vi "Test App Broadcast Nested Process Messages.vi"(8 "error in (no error)":errorcluster, 11 "Application Test In":refnum<class "Application Dev Test.lvclass">) -> (0 "error out":errorcluster, 3 "Application Test Out":refnum<class "Application Dev Test.lvclass">)   [LabVIEW 2020, in "Application Dev Test.lvclass"]
uses:
  Application Dev Test.lvclass
  C:/Program Files (x86)/National Instruments/LabVIEW 2020/vi.lib/Astemes/LUnit/Test Case.lvclass
  source/Framework Test Suite/Mock Process/Mock Process.lvclass
  C:/Git/astemes-triarc-framework/source/Framework/Process/Process.lvclass
  source/Framework/Application/Application.lvclass
  source/Framework/Process/Process.lvclass/Process.ctl
  source/Framework/Application/Application.lvclass/Application.ctl
  <vilib>/Astemes/LUnit/Test Case.lvclass/Test Case.ctl
  c27f4279-7cb7-4f54-8dc5-63ff7bac36e5.vi
  76411ce1-69dc-435f-b6fb-e9cd8e6b3fac.vi
  source/Framework/Application/Private/Add Process to Map.vi
  source/Framework/Application/Private/Throw Error If Process Already in App.vi
  source/Framework/Process/Protected/Messaging/Send Message.vi
  source/Framework/Process/Public/Lifecycle/Get Lifecycle State.vi
  source/Framework/Process/Protected/SubVIs/Set Context.vi
  source/Framework/Process/Private/SubVIs/Wait for finish.vi
  source/Framework/Process/Private/SubVIs/Set Lifecycle State.vi
  source/Framework/Broadcast Event Helpers/Execution timer.vi
  <vilib>/Astemes/LUnit/Palette/Pass.vi
  <vilib>/Astemes/LUnit/Palette/Fail.vi
  <vilib>/Astemes/LUnit/Compare Variants.vi
  <vilib>/Astemes/LUnit/Describe Comparison.vi
  <vilib>/Astemes/LUnit/Set Assertion Type.vi
  source/Framework/Application/Public/Get Process.vi
  source/Framework/Process/Private/SubVIs/Handle Debug Data.vi
  <vilib>/Utility/error.llb/Clear Errors.vi
  source/Framework/Process/Public/Lifecycle/Leave Process Loop.vi
  <vilib>/Astemes/LUnit/Add test result.vi
  <vilib>/Astemes/LUnit/Variant to string.vi
  source/Framework/Application/Private/Retrieve Process from App.vi
  source/Framework/Application/Private/Parse Process Name.vi
  source/Framework/Application/Private/Get Process from Map.vi
  source/Framework/Logging/Log Debug.vi
  <vilib>/AdvancedString/1D String Array to Delimited String.vi
  <vilib>/Utility/High Resolution Relative Seconds.vi
  <vilib>/Astemes/LUnit/LUnit Record Assertion Result.vi
  source/Framework/Process/Protected/Messaging/Request Message.vi
  <vilib>/AdvancedString/Delimited String to 1D String Array.vi
  <vilib>/Astemes/LUnit/LUnit Aggregate Assertion Results.vi
  source/Framework/Process/Private/SubVIs/Enqueue Request Message.vi
  <vilib>/Astemes/LUnit/Method Result/LUnit Merge Status.vi
  <vilib>/Astemes/LUnit/LUnit Concatenate result strings.vi
  <vilib>/Utility/error.llb/Error Cluster From Error Code.vi
  source/Framework/Process/Public/Read Name.vi
  source/Framework/Process/Private/SubVIs/Wait for Response Message.vi
  source/Framework/Application/Protected/Get Broadcast Events Recursively.vi
  source/Framework/Broadcast Event Helpers/Dequeue Broadcast Message.vi
  <vilib>/Utility/Data Type/Get Type Information.vi
  <vilib>/Utility/LVClass/Get LV Class Name.vi
  source/Framework/Process/Process.lvclass
  Application Dev Test.lvclass/Application Dev Test.ctl
  C:/Git/astemes-triarc-framework/source/Framework/Base/Base.lvclass
  C:/Git/astemes-triarc-framework/source/Framework/Configuration File/Configuration File.lvclass
  C:/Git/astemes-triarc-framework/source/Framework/Configuration/Configuration.lvclass
  C:/Git/astemes-triarc-framework/source/Framework/Error Handler Interface/Error Handler Interface.lvclass
  C:/Git/astemes-triarc-framework/source/Framework/Logging/Logging.lvclass
  C:/Git/astemes-triarc-framework/source/Framework Test Suite/Mock Process/Mock Process.lvclass
  C:/Git/astemes-triarc-framework/source/Framework/Async Handler/Async Handler.lvclass
  C:/Git/astemes-triarc-framework/source/Framework/Helper Loop/Helper Loop.lvclass
  C:/Git/astemes-triarc-framework/source/Framework/Application/Application.lvclass
  source/Framework/Broadcast Event Helpers/Broadcast Event Helpers.lvlib
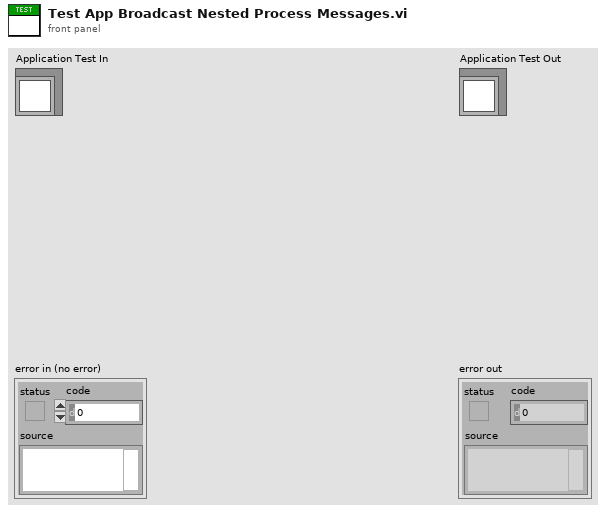
[diagram p1: front panel]
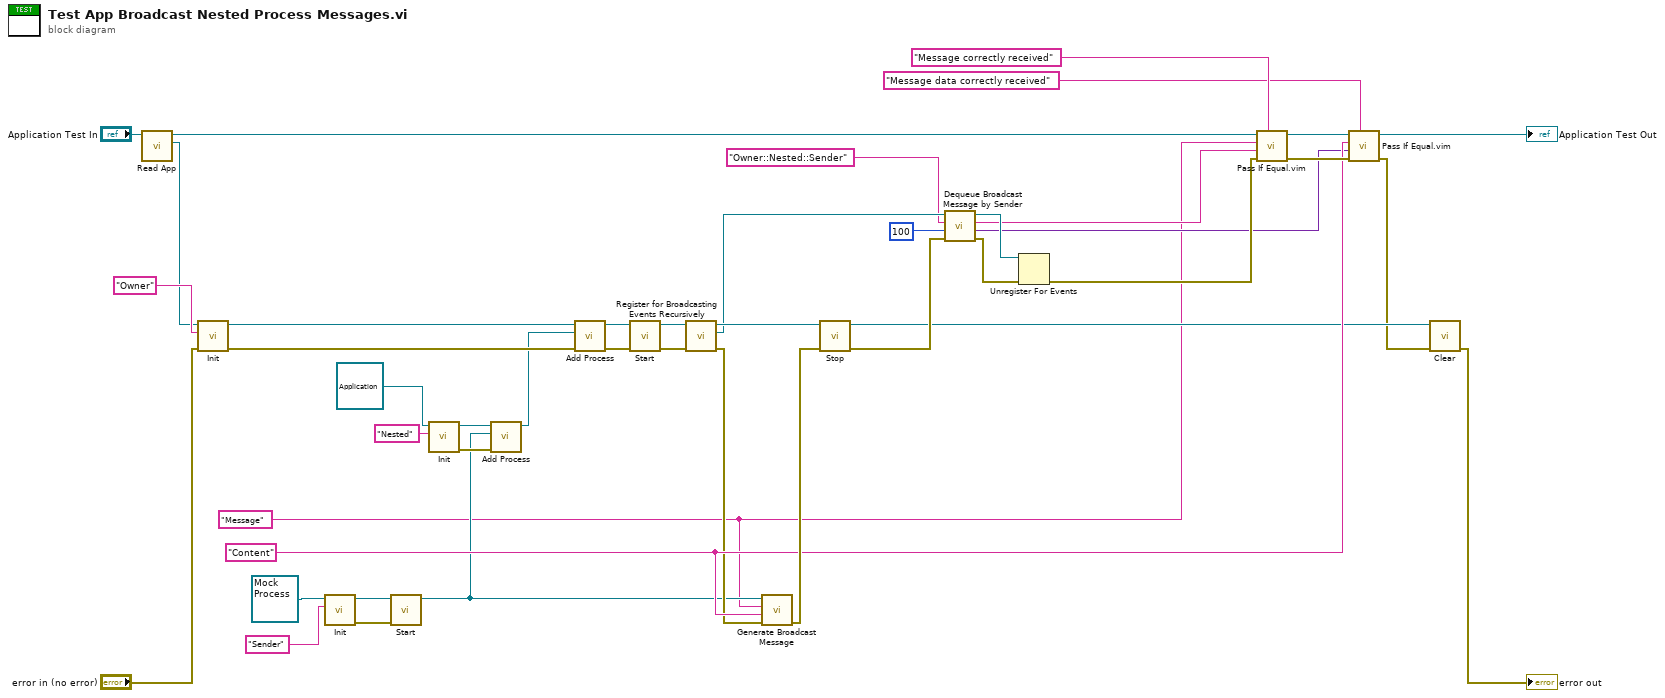
[diagram p0: block diagram]
diagram:
  w23 = "Content" ("Message")
  w1 = "Message" ("Message")
  n1 = call "Read App.vi"("Application Test In"="Application Test In") -> ("App out"=w26:refnum<class "Application.lvclass">, "Application Test Out"=w27:refnum<class "Application Dev Test.lvclass">)  [unwired: 8 in, 1 out]
  n2 = call-dynamic "Init.vi"("error in (no error)"="error in (no error)", "Name"="Owner" ("Message"), "Process In"=w26) -> ("error out"=w42:errorcluster, "Process Out"=w43:refnum<class "Application.lvclass">)  [unwired: 7 in]
  n3 = call-dynamic "Init.vi"("Name"="Sender" ("Message"), "Mock Process In"=refnum<class "Mock Process.lvclass"> refnum ("Mock Process.lvclass")) -> ("error out"=w30:errorcluster, "Mock Process Out"=w29:refnum<class "Mock Process.lvclass">)  [unwired: 8 in]
  n4 = call "Start.vi"("error in (no error)"=w30, "Process In"=w29) -> ("Process Out"=w8:refnum<class "Mock Process.lvclass">)  [unwired: 7 in, 2 out]
  n5 = call-dynamic "Init.vi"("Name"="Nested", "Process In"=refnum<class "Application.lvclass"> refnum ("Process Out")) -> ("error out"=w11:errorcluster, "Process Out"=w10:refnum<class "Application.lvclass">)  [unwired: 8 in]
  n6 = call "Add Process.vi"("error in (no error)"=w11, "Process"=w8, "Application In"=w10) -> ("Application Out"=w7:refnum<class "Application.lvclass">)  [unwired: 7 in, 1 out]
  n7 = call "Add Process.vi"("error in (no error)"=w42, "Process"=w7, "Application In"=w43) -> ("error out"=w18:errorcluster, "Application Out"=w3:refnum<class "Application.lvclass">)  [unwired: 7 in]
  n8 = call "Start.vi"("error in (no error)"=w18, "Process In"=w3) -> ("error out"=w4:errorcluster, "Process Out"=w2:refnum<class "Application.lvclass">)  [unwired: 7 in, 1 out]
  n9 = call "Register for Broadcasting Events Recursively.vi"("error in (no error)"=w4, "Application In"=w2) -> ("error out"=w16:errorcluster, "Event Registration Refnum Out"=w15:refnum<event-registration>, "Application Out"=w17:refnum<class "Application.lvclass">)  [unwired: 7 in]
  n10 = call "Generate Broadcast Message.vi"("error in (no error)"=w16, "Message Data"=w23, "Message"=w1, "Mock Process In"=w8) -> ("error out"=w25:errorcluster)  [unwired: 6 in, 1 out]
  n11 = call "Stop.vi"("error in (no error)"=w25, "Process In"=w17) -> ("error out"=w41:errorcluster, "Process Out"=w14:refnum<class "Application.lvclass">)  [unwired: 7 in, 1 out]
  n12 = call "Dequeue Broadcast Message by Sender.vi"("error in (no error)"=w41, "Timeout (-1)"=100, "Sender"="Owner::Nested::Sender" ("Message"), "Event Registration Refnum"=w15) -> ("error out"=w19:errorcluster, "Message Data"=w21:variant, "Message"=w22:string, "Event Registration Refnum Out"=w39:refnum<event-registration>)  [unwired: 3 in, 1 out]
  n13 = Unregister For Events(event registration refnum=w39, error in=w19) -> (error out=w35:errorcluster)
  n14 = call "Pass If Equal.vim"("Description"="Message correctly received", "error in (no error)"=w35, "Actual"=w22, "Expected"=w1, "LUnit Test Case In"=w27) -> ("error out"=w36:errorcluster, "LUnit Test Case Out"=w37:refnum<class "Application Dev Test.lvclass">)  [unwired: 5 in]
  n15 = call "Pass If Equal.vim"("Description"="Message data correctly received", "error in (no error)"=w36, "Actual"=w21, "Expected"=w23, "LUnit Test Case In"=w37) -> ("error out"=w13:errorcluster, "LUnit Test Case Out"=→"Application Test Out":refnum<class "Application Dev Test.lvclass">)  [unwired: 5 in]
  n16 = call-dynamic "Clear.vi"("error in (no error)"=w13, "Application In"=w14) -> ("error out"=→"error out":errorcluster)  [unwired: 9 in]
